vi "Billard2020.vi"() -> ()   [LabVIEW 2019]
panel:
  in  "Sequence":path
  in  "Enable image":bool=TRUE
  in  "Execute matlab script":bool=TRUE
  in  "Compilation":T1(ring)
  in  "Advanced control":T2={"RedBall"={"Min"={"G"=0, "B"=0, "R"=160}, "Max"={"G"=160, "B"=160, "R"=255}}, "YellowBall"={"Min"={"G"=140, "B"=0, "R"=140}, "Max"={"G"=255, "B"=175, "R"=255}}, "WhiteBall"={"Min"={"G"=100, "B"=100, "R"=100}, "Max"={"G"=255, "B"=255, "R"=255}}, "BallDiameter"=11, "BackGround"={"Min"={"G"=91, "B"=202, "R"=39}, "Max"={"G"=116, "B"=255, "R"=62}}, "Border"={"Min"={"G"=0, "B"=121, "R"=0}, "Max"={"G"=42, "B"=126, "R"=14}}}
  in  "Select line style":string(combo)=" -"
  in  "Ball touch color":u32(colorbox)=6618880
  in  "Band touch color":u32(colorbox)=3381759
  out "current frame":picture
  out "frame num":i32
  out "error out":errorcluster
  in  "error in (no error)":errorcluster
  # "Style control"
  # "Frame display"
  # "Functional control"
  # "Error reports"
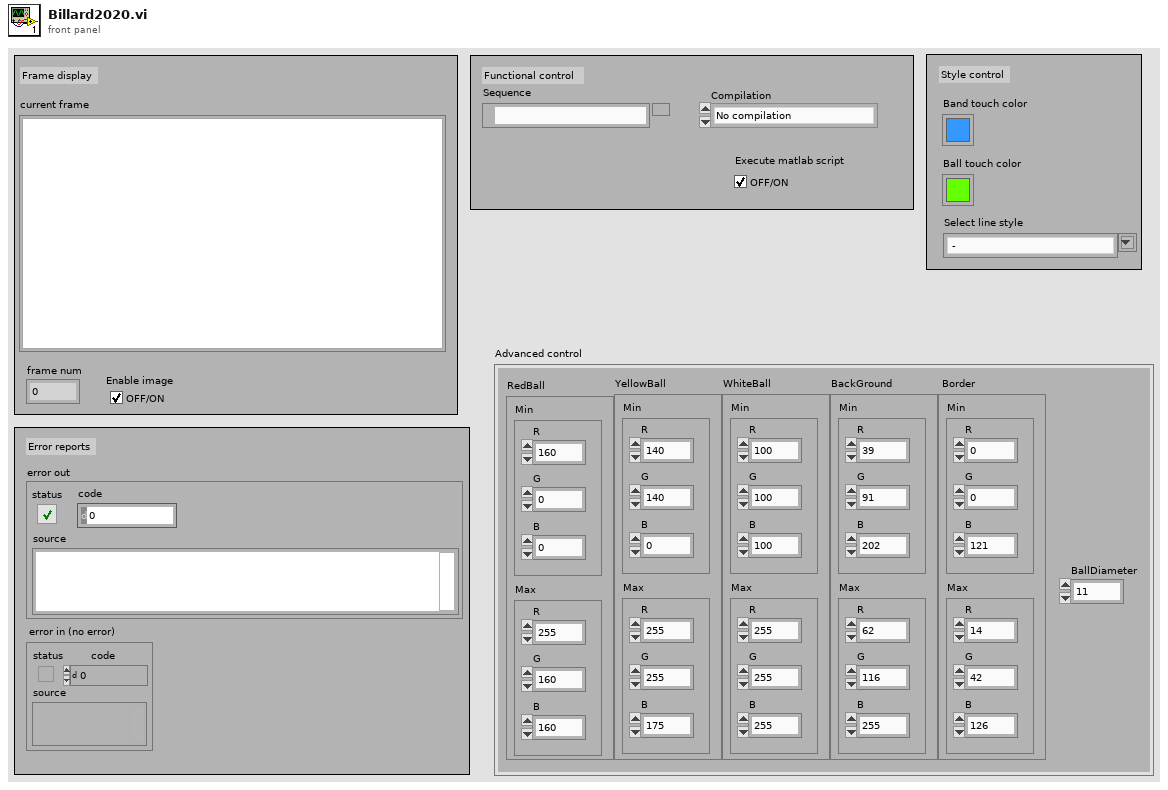
[diagram p1: front panel]
types:
  T1 = enum16{"No compilation", "No memory", "With memory", "Simple"}
  T2 = cluster{"RedBall":cluster{"Min":cluster{"G":u32, "B":u32, "R":u32}, "Max":cluster{"G":u32, "B":u32, "R":u32}}, "YellowBall":cluster{"Min":cluster{"G":u32, "B":u32, "R":u32}, "Max":cluster{"G":u32, "B":u32, "R":u32}}, "WhiteBall":cluster{"Min":cluster{"G":u32, "B":u32, "R":u32}, "Max":cluster{"G":u32, "B":u32, "R":u32}}, "BallDiameter":u32, "BackGround":cluster{"Min":cluster{"G":u32, "B":u32, "R":u32}, "Max":cluster{"G":u32, "B":u32, "R":u32}}, "Border":cluster{"Min":cluster{"G":u32, "B":u32, "R":u32}, "Max":cluster{"G":u32, "B":u32, "R":u32}}}
  T3 = cluster{"Red":cluster{"X":u32, "Y":u32, "Score":u32}, "Yellow":cluster{"X":u32, "Y":u32, "Score":u32}, "White":cluster{"X":u32, "Y":u32, "Score":u32}}[]
  T4 = cluster{"Red":cluster{"X":u32, "Y":u32, "Score":u32}, "Yellow":cluster{"X":u32, "Y":u32, "Score":u32}, "White":cluster{"X":u32, "Y":u32, "Score":u32}}
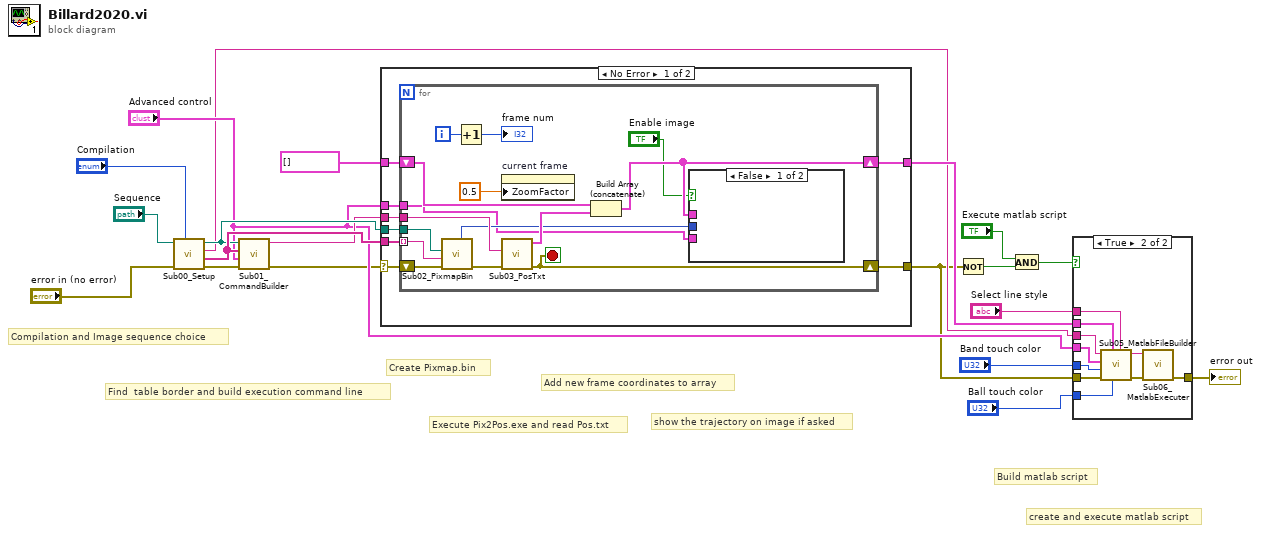
[diagram p0: block diagram]
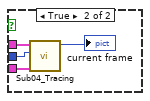
[diagram p3: hidden frame]
diagram:
  # "create and execute matlab script"
  # "Build matlab script"
  # "show the trajectory on image if asked"
  # "Add new frame coordinates to array"
  # "Execute Pix2Pos.exe and read Pos.txt"
  # "Create Pixmap.bin"
  # "Find  table border and build execution command line"
  # "Compilation and Image sequence choice"
  n1 = call "Sub00_Setup.vi"("Enum"="Compilation", "error in (no error)"="error in (no error)", "Sequence"="Sequence") -> ("error out"=w18:errorcluster, "filenames"=w20:string[], "name"=w8:string, "path out"=w19:path)  [unwired: 5 in]
  n2 = call "Sub01_CommandBuilder.vi"("error in (no error)"=w18, "CommandInfo"="Advanced control", "filenames"=w20, "path in"=w19) -> ("error out"=w1:errorcluster, "String"=w16:string)  [unwired: 6 in]
  n3 = case shown="No Error" w1 {
    selector: w1 -> [w23 w49]
    tunnel: w19 -> [w28 _]
    tunnel: w20 -> [w27 _]
    tunnel: [w22 w49] -> w2
    tunnel: w16 -> [w26 _]
    tunnel: [w25 w48] -> w12
    tunnel: T3 [] ("appended array") -> [w24 w48]
    tunnel: "Advanced control" -> [w21 _]
    frame No Error {
      n4 = for {
        tunnel: w28 -> [w43]
        tunnel: w27 -> [w42] mode=indexing
        tunnel: w26 -> [w40]
        shift-right: [w34] -> w25
        shift-left: w24 -> [w38]
        shift-right: [w30] -> w22
        shift-left: w23 -> [w33]
        tunnel: w21 -> [w31]
        i -> [w39]
        stop <- w30 stop-if-true
        n5 = call "Sub02_PixmapBin.vi"("error in (no error)"=w33, "String"=w42, "path in"=w43) -> ("error out"=w41:errorcluster, "new picture"=w35:picture)  [unwired: 7 in]
        n6 = Increment(x=w39) -> (x+1=→"frame num":i32)
        n7 = property on="current frame" class="Pict"("ZoomFactor"=sgl 0.5 ("Zoom Factor")) -> ()  [unwired: 2 in, 2 out]
        n8 = call "Sub03_PosTxt.vi"("error in (no error)"=w41, "String"=w40) -> ("error out"=w30:errorcluster, "output cluster"=w36:T4)  [unwired: 6 in, 2 out]
        n9 = Build Array (concatenate)(w38, w36) -> (w34:T3)
        n10 = case shown="False" "Enable image" {
          tunnel: w35 -> [_ w47]
          tunnel: w34 -> [_ w46]
          tunnel: w31 -> [_ w45]
          frame False {
          }
          frame True {
            n11 = call "Sub04_Tracing.vi"("CommandInfo"=w45, "new picture in"=w47, "Array"=w46) -> ("new picture out"=→"current frame":picture)  [unwired: 8 in]
          }
        }
      }
    }
    frame Error {
    }
  }
  n12 = Not(x=w2) -> (.not. x?=w3:bool)
  n13 = And(x="Execute matlab script", y=w3) -> (x .and. y?=w4:bool)
  n14 = case shown="True" w4 {
    tunnel: w2 -> [w50 w60]
    tunnel: "Band touch color" -> [_ w59]
    tunnel: "Ball touch color" -> [_ w58]
    tunnel: "Select line style" -> [_ w57]
    tunnel: w12 -> [_ w56]
    tunnel: [w50 w53] -> w11
    tunnel: "Advanced control" -> [_ w52]
    tunnel: w8 -> [_ w51]
    frame False {
    }
    frame True {
      n15 = call "Sub05_MatlabFileBuilder.vi"("Select line style"=w57, "Ball touch color"=w58, "appended array"=w56, "error in (no error)"=w60, "Band touch color"=w59, "CommandInfo"=w52, "Select sequence"=w51) -> ("error out"=w54:errorcluster, "Script"=w55:string)  [unwired: 3 in]
      n16 = call "Sub06_MatlabExecuter.vi"("error in (no error)"=w54, "Script"=w55) -> ("error out"=w53:errorcluster)  [unwired: 7 in, 2 out]
    }
  }
  "error out" <- w11
